vi "codificare.vi"() -> ()   [LabVIEW 2019]
panel:
  out "String 2":string
  in  "String":string
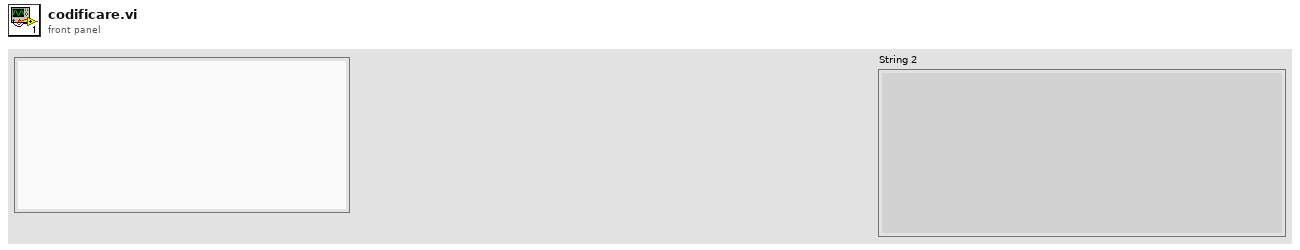
[diagram p1: front panel]
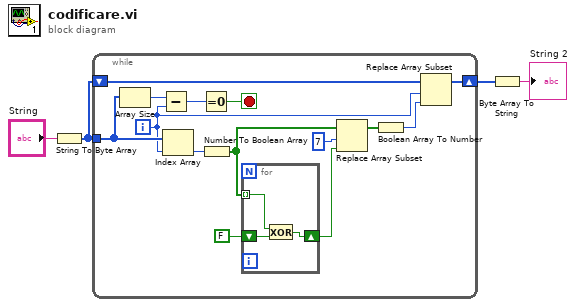
[diagram p0: block diagram]
diagram:
  n1 = String To Byte Array(string="String") -> (unsigned byte array=w3:u8[])
  n2 = while {
    tunnel: w3 -> [w18]
    shift-right: [w8] -> w2
    shift-left: w3 -> [w7]
    i -> [w6]
    stop <- w15 stop-if-true
    n3 = Array Size(array=w18) -> (size(s)=w17:i32)
    n4 = Subtract(x=w17, y=w6) -> (x-y=w16:i32)
    n5 = Index Array(array=w18, index=w6) -> (element=w10:u8)
    n6 = Equal To 0?(x=w16) -> (x = 0?=w15:bool)
    n7 = Number To Boolean Array(number=w10) -> (Boolean array=w12:bool[])
    n8 = for {
      tunnel: w12 -> [w19] mode=indexing
      shift-right: [w20] -> w13
      shift-left: FALSE -> [w21]
      n9 = Exclusive Or(1:w21, 2:w19) -> (0:w20:bool)
    }
    n10 = Replace Array Subset(array=w12, new element=w13, index=7) -> (w9:bool[])
    n11 = Boolean Array To Number(Boolean array=w9) -> (number=w5:u32)
    n12 = Replace Array Subset(array=w7, new element=w5, index=w6) -> (w8:u8[])
  }
  n13 = Byte Array To String(unsigned byte array=w2) -> (string=→"String 2":string)
